vi "McLeod's Estimator Interpolation method.vi"(11 "FFT array":dbl[](array[numeric])) -> (0 "max index(es)":i32, 3 "Index Bin":dbl)   [LabVIEW 2014]
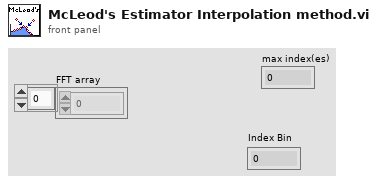
[diagram p1: front panel]
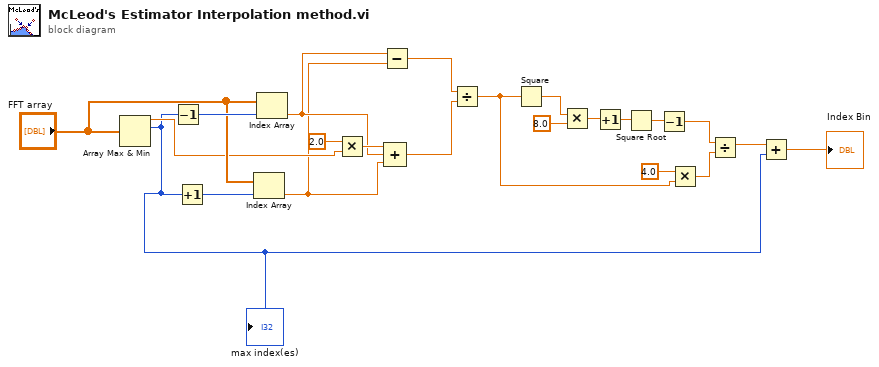
[diagram p0: block diagram]
diagram:
  n1 = Array Max & Min(array="FFT array") -> (max value=w18:dbl, max index (indices)=w2:i32)  [unwired: 2 out]
  "max index(es)" <- w2
  n2 = Decrement(x=w2) -> (x-1=w22:i32)
  n3 = Increment(x=w2) -> (x+1=w21:i32)
  n4 = Index Array(array="FFT array", index=w21) -> (element=w15:dbl)
  n5 = Index Array(array="FFT array", index=w22) -> (element=w16:dbl)
  n6 = Multiply(x=2.0, y=w18) -> (x*y=w17:dbl)
  n7 = Subtract(x=w16, y=w15) -> (x-y=w13:dbl)
  n8 = Compound Arithmetic op=ADD(w17, w16, w15) -> (w14:dbl)
  n9 = Divide(x=w13, y=w14) -> (x/y=w6:dbl)
  n10 = Square(x=w6) -> (x^2=w12:dbl)
  n11 = Multiply(x=w12, y=8.0) -> (x*y=w10:dbl)
  n12 = Increment(x=w10) -> (x+1=w9:dbl)
  n13 = Square Root(x=w9) -> (sqrt(x)=w8:dbl)
  n14 = Decrement(x=w8) -> (x-1=w5:dbl)
  n15 = Multiply(x=4.0, y=w6) -> (x*y=w4:dbl)
  n16 = Divide(x=w5, y=w4) -> (x/y=w3:dbl)
  n17 = Add(x=w3, y=w2) -> (x+y=→"Index Bin":dbl)
